vi "Set Params.vi"(8 "error in (no error)":errorcluster, 10 "CoordinatesIN":T1 {"Z" step=10.0}, 11 "reference in":refnum<class "Manipulator.lvclass">) -> (0 "error out":errorcluster, 3 "reference out":refnum<class "Manipulator.lvclass">)   [LabVIEW 2014, in "Manipulator.lvclass"]
uses:
  Manipulator.lvclass
  typedefs/Coordinates.ctl
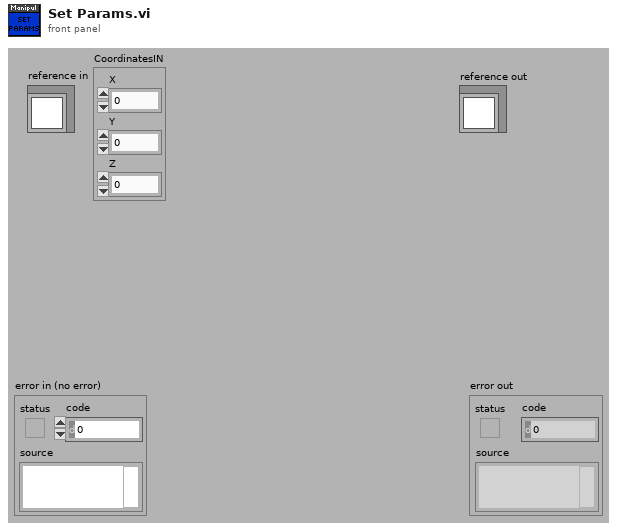
[diagram p1: front panel]
types:
  T1 = typedef "Manipulator.lvclass/Coordinates.ctl" = cluster{"X":dbl, "Y":dbl, "Z":dbl}
  T2 = typedef "Manipulator.lvclass/ObjectAttributes.ctl" = cluster{"Coordinates":cluster{"X":dbl, "Y":dbl, "Z":dbl}, "Angles":cluster{"THETA_1":dbl, "THETA_2":dbl, "THETA_3":dbl, "THETA_4":dbl, "THETA_5":dbl, "THETA_6":dbl, "THETA_7":dbl, "THETA_8":dbl, "THETA_9":dbl, "THETA_10":dbl}, "Lengths":cluster{"a":dbl, "b":dbl, "c":dbl, "d":dbl, "e":dbl}, "Coordinates of joints":cluster{"A":cluster{"X":dbl, "Y":dbl, "Z":dbl}, "B":cluster{"X":dbl, "Y":dbl, "Z":dbl}, "C":cluster{"X":dbl, "Y":dbl, "Z":dbl}, "D":cluster{"X":dbl, "Y":dbl, "Z":dbl}}}
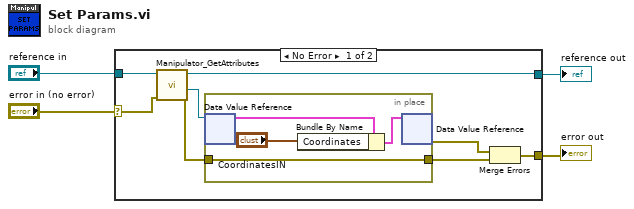
[diagram p0: block diagram]
diagram:
  n1 = case shown="No Error" "error in (no error)" {
    selector: "error in (no error)" -> [w11 w18]
    tunnel: [w8 w18] -> w3
    tunnel: [w9 w17] -> w1
    tunnel: "reference in" -> [w12 w17]
    frame No Error {
      n2 = call "Manipulator_GetAttributes.vi"("error in (no error)"=w11, "reference in"=w12) -> ("error out"=w6:errorcluster, "DataRef"=w7:refnum<data-value>, "reference out"=w9:refnum<class "Manipulator.lvclass">)  [unwired: 6 in, 1 out]
      n3 = in-place {
        in-place-border: w6 -> [w16]
        in-place-border: [w16] -> w5
        n4 = in-place-dvr #1(w7) -> (w15:T2)  [unwired: 1 out]
        n5 = Bundle By Name(cluster=w15, "Coordinates"="CoordinatesIN") -> (w14:T2)
        n6 = in-place-dvr #1(w14) -> (w10:errorcluster)  [unwired: 1 out]
      }
      n7 = Merge Errors(w10, w5) -> (w8:errorcluster)
    }
    frame Error {
    }
  }
  "error out" <- w3
  "reference out" <- w1
